vi "entityLoop.vi"() -> ()   [LabVIEW 2012]
uses:
  <vilib>/Utility/file.llb/Read From Spreadsheet File (string).vi
panel:
  out "before substring":string
  out "element":string
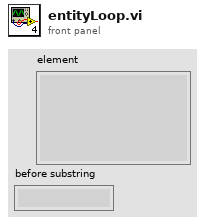
[diagram p1: front panel]
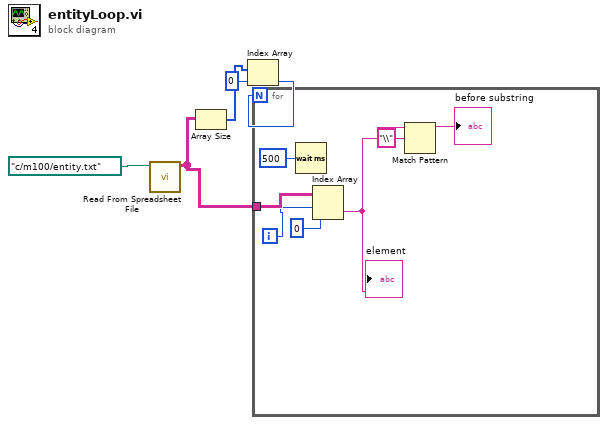
[diagram p0: block diagram]
diagram:
  n1 = call-poly <vilib>:"Read From Spreadsheet File.vi"("file path (dialog if empty)"=path "c:/m100/entity.txt" ("file path (use dialog)")) -> ("all rows"=w4:string[][])  [unwired: 6 in, 4 out]
  n2 = Array Size(array=w4) -> (size(s)=w3:i32[])
  n3 = Index Array(array=w3, index=0) -> (element=w1:i32)
  n4 = for {
    N: w1 -> [_]
    tunnel: w4 -> [w12]
    i -> [w10]
    n5 = Wait (ms)(milliseconds to wait=u32 500) -> ()  [unwired: 1 out]
    n6 = Index Array(array=w12, index (row)=w10, index (col)=0 ("disabled index (col)")) -> (element=w8:string)
    "element" <- w8
    n7 = Match Pattern(string=w8, regular expression="\\") -> (before substring=→"before substring":string)  [unwired: 1 in, 3 out]
  }
